vi "ExternalVIDefaultSave.vi"(10 "Control2SetDefault":string[](array[string]), 11 "VI in":refnum<vi>) -> ()   [LabVIEW 2020]
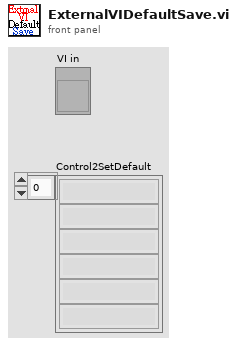
[diagram p1: front panel]
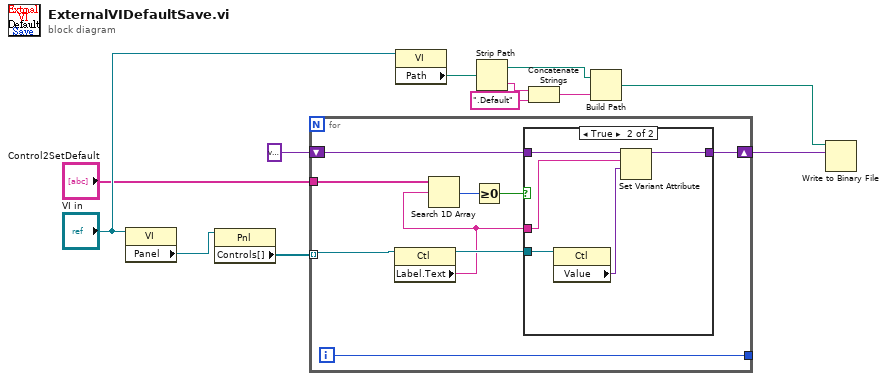
[diagram p0: block diagram]
diagram:
  n1 = property class="VI"(reference="VI in") -> ("Panel"=w4:refnum<vi>)  [unwired: 1 in, 2 out]
  n2 = property class="Pnl"(reference=w4) -> ("Controls[]"=w3:refnum<vi>[])  [unwired: 1 in, 2 out]
  n3 = for {
    tunnel: w3 -> [w20] mode=indexing
    tunnel: "Control2SetDefault" -> [w21]
    shift-right: [w14] -> w12
    shift-left: variant -> [w15]
    tunnel: [w13] -> _
    i -> [w13]
    n4 = property class="Ctl"(reference=w20) -> (reference out=w17:refnum<vi>, "Label.Text"=w16:string)  [unwired: 1 in, 1 out]
    n5 = Search 1D Array(1D array=w21, element=w16) -> (index of element=w19:i32)  [unwired: 1 in]
    n6 = Greater Or Equal To 0?(x=w19) -> (x >= 0?=w18:bool)
    n7 = case shown="True" w18 {
      tunnel: w17 -> [_ w27]
      tunnel: w16 -> [_ w25]
      tunnel: w15 -> [w22 w26]
      tunnel: [w22 w23] -> w14
      frame False {
      }
      frame True {
        n8 = property class="Ctl"(reference=w27) -> ("Value"=w24:variant)  [unwired: 1 in, 2 out]
        n9 = Set Variant Attribute(Variant=w26, name=w25, value=w24) -> (Variant out=w23:variant)  [unwired: 1 in, 2 out]
      }
    }
  }
  n10 = property class="VI"(reference="VI in") -> ("Path"=w6:path)  [unwired: 1 in, 2 out]
  n11 = Strip Path(path=w6) -> (stripped path=w9:path, name=w7:string)
  n12 = Concatenate Strings(w7, ".Default" ("string")) -> (w10:string)
  n13 = Build Path(base path=w9, name or relative path=w10) -> (appended path=w11:path)
  n14 = Write to Binary File(file (use dialog)=w11, data=w12) -> ()  [unwired: 4 in, 3 out]
